vi "Facade.vi"(0 "Data In":T4, 2 "Display State In":T2, 3 "Container State":T3) -> (6 "Data Out":T4, 7 "Display State Out":T2, 8 "Action":T1)   [LabVIEW 2015, in "KCheckbox.xctl"]
uses:
  KCheckbox.xctl
  Data.ctl
  <vilib>/_xctls/Container State.ctl
  State.ctl
  <vilib>/_xctls/Action.ctl
  <vilib>/_xctls/XControlSupport.lvlib
panel:
  in  "Checkbox":enum8{"False", "True", "Mixed"}(c332)
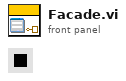
[diagram p1: front panel]
types:
  T1 = typedef "XControlSupport.lvlib/Action.ctl" = cluster{"Data Changed?":bool, "State Changed?":bool, "Action Name":string}
  T2 = typedef "KCheckbox.xctl/State.ctl" = cluster{"mixed":bool, "Value":bool, "update":bool}
  T3 = typedef "XControlSupport.lvlib/Container State.ctl" = cluster{"Indicator?":bool, "Run Mode?":bool, " Refnum":refnum<vi>}
  T4 = typedef "KCheckbox.xctl/Data.ctl" = bool
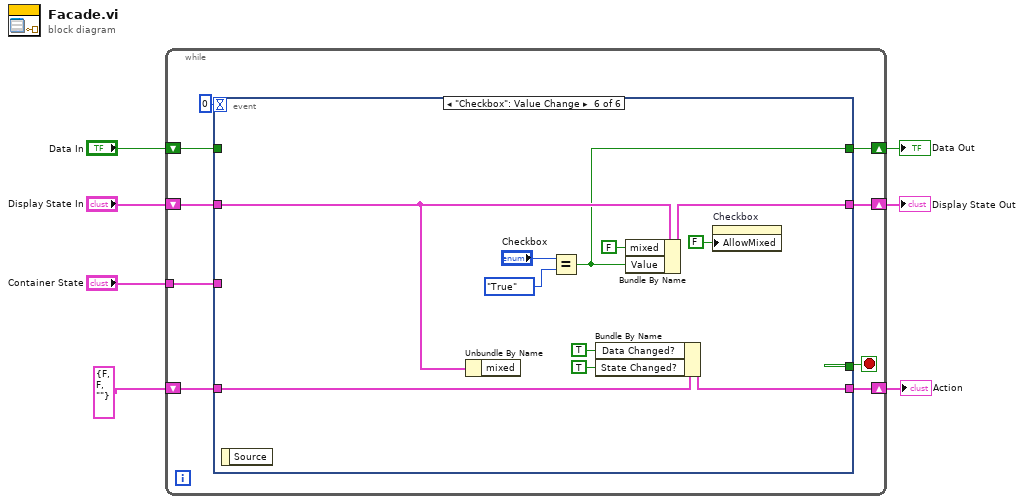
[diagram p0: block diagram]
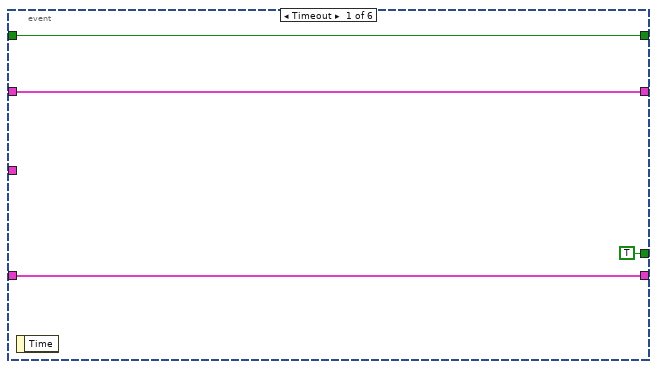
[diagram p2: hidden frame]
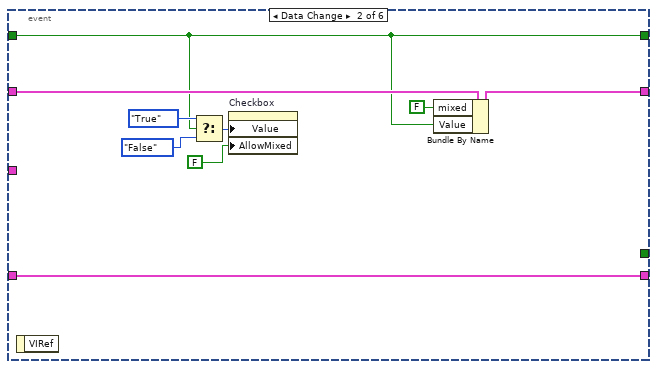
[diagram p3: hidden frame]
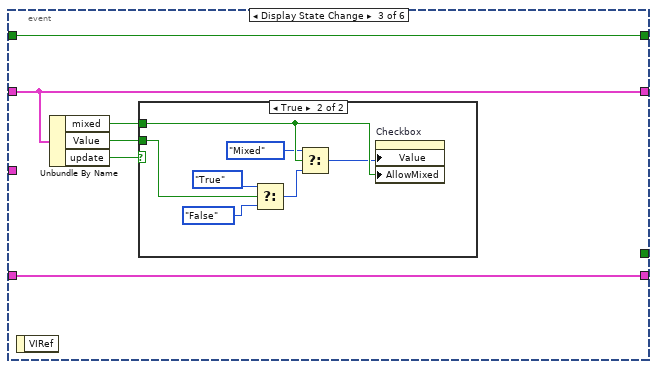
[diagram p4: hidden frame]
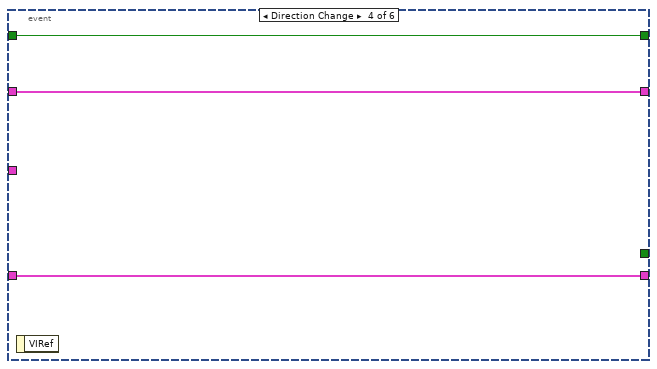
[diagram p6: hidden frame]
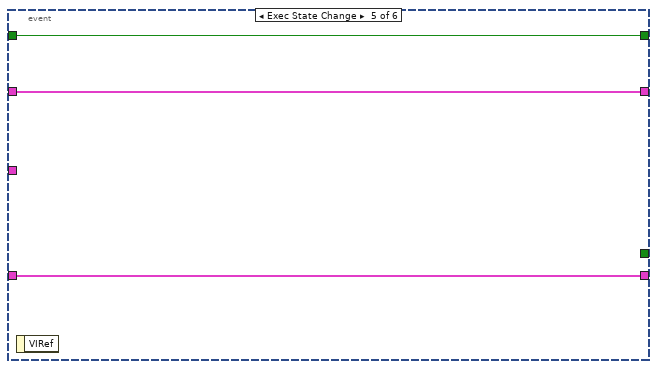
[diagram p7: hidden frame]
diagram:
  n1 = while {
    shift-right: [w15] -> w4
    shift-left: "Display State In" -> [w16]
    tunnel: "Container State" -> [w12]
    shift-right: [w10] -> w7
    shift-left: "Data In" -> [w11]
    shift-right: [w8] -> w2
    shift-left: T1 {"Data Changed?"=FALSE, "State Changed?"=FALSE, "Action Name"=""} ("Action") -> [w9]
    stop <- w14 stop-if-true
    n2 = event shown="[5] \"Checkbox\": Value Change" {
      selector: _ -> [_ _ _ _ _ _]
      dyn-events: _ -> [_ _ _ _ _ _]
      timeout: 0 -> [_ _ _ _ _ _]
      tunnel: w16 -> [w18 w29 w33 w43 w48 w53]
      tunnel: [w18 w23 w33 w43 w48 w58] -> w15
      tunnel: [TRUE _ _ _ _ _] -> w14
      tunnel: w12 -> [_ _ _ _ _ _]
      tunnel: w11 -> [w17 w21 w32 w44 w47 _]
      tunnel: [w17 w21 w32 w44 w47 w50] -> w10
      tunnel: [w19 w28 w35 w45 w46 w56] -> w8
      tunnel: w9 -> [w19 w28 w35 w45 w46 w59]
      event Timeout {
        n3 = event-data() -> ()  [unwired: 1 in, 1 out]
      }
      event Data Change {
        n4 = event-data() -> ()  [unwired: 1 in, 1 out]
        n5 = Select(t=enum8{"False", "True", "Mixed"}."True", s=w21, f=enum8{"False", "True", "Mixed"}."False" ("Checkbox")) -> (s? t:f=w27:enum8{"False", "True", "Mixed"})
        n6 = property on="Checkbox" class="MixedCheckbox (strict)"("Value"=w27, "AllowMixed"=FALSE ("Allow Mixed")) -> ()  [unwired: 2 in, 2 out]
        n7 = Bundle By Name(cluster=w29, "mixed"=FALSE, "Value"=w21) -> (w23:T2)
      }
      event Display State Change {
        n8 = event-data() -> ()  [unwired: 1 in, 1 out]
        n9 = Unbundle By Name(w33) -> ("mixed"=w34:bool, "Value"=w31:bool, "update"=w30:bool)
        n10 = case shown="True" w30 {
          tunnel: w34 -> [_ w40]
          tunnel: w31 -> [_ w36]
          frame False {
          }
          frame True {
            n11 = Select(t=enum8{"False", "True", "Mixed"}."True", s=w36, f=enum8{"False", "True", "Mixed"}."False" ("Checkbox")) -> (s? t:f=w39:enum8{"False", "True", "Mixed"})
            n12 = Select(t=enum8{"False", "True", "Mixed"}."Mixed", s=w40, f=w39) -> (s? t:f=w37:enum8{"False", "True", "Mixed"})
            n13 = property on="Checkbox" class="MixedCheckbox (strict)"("Value"=w37, "AllowMixed"=w40) -> ()  [unwired: 2 in, 2 out]
          }
        }
      }
      event Direction Change {
        n14 = event-data() -> ()  [unwired: 1 in, 1 out]
      }
      event Exec State Change {
        n15 = event-data() -> ()  [unwired: 1 in, 1 out]
      }
      event "Checkbox": Value Change {
        n16 = event-data() -> ()  [unwired: 1 in, 1 out]
        n17 = Unbundle By Name(w53) -> ()  [unwired: 1 out]
        n18 = Equal?(x="Checkbox", y=enum8{"False", "True", "Mixed"}."True") -> (x = y?=w50:bool)
        n19 = Bundle By Name(cluster=w59, "Data Changed?"=TRUE, "State Changed?"=TRUE) -> (w56:T1)
        n20 = Bundle By Name(cluster=w53, "mixed"=FALSE, "Value"=w50) -> (w58:T2)
        n21 = property on="Checkbox" class="MixedCheckbox (strict)"("AllowMixed"=FALSE ("Allow Mixed")) -> ()  [unwired: 2 in, 2 out]
      }
    }
  }
  "Display State Out" <- w4
  "Data Out" <- w7
  "Action" <- w2
